vi "Receive Value Change Event.vi"(8 "error in (no error)":errorcluster, 10 "ValueChangeMsg":refnum<class "ValueChangeMsg.lvclass">, 11 "TwoButtonDialogBox in":refnum<class "TwoButtonDialogBox.lvclass">) -> (0 "error out":errorcluster, 3 "TwoButtonDialogBox out":refnum<class "TwoButtonDialogBox.lvclass">)   [LabVIEW 2017, in "TwoButtonDialogBox.lvlib" / "TwoButtonDialogBox.lvclass"]
doc: "<License>\nCopyright © 2017 Composed Systems, LLC | All rights reserved\nwww.composed.io\n\nAuthor: Ethan Stern <ethan.stern@composed.io>\n\nThis software is provided \"AS IS\" WITHOUT WARRANTIES, either express or implied, AND IS FOR EDUCATIONAL PURPOSES ONLY.\n</License>"
uses:
  TwoButtonDialogBox.lvclass
  C:/Program Files (x86)/National Instruments/LabVIEW 2017/vi.lib/ActorFramework/Actor/Actor.lvclass
  Framework/ActorEvents/IEventAggregator Messages/ValueChangeMsg/ValueChangeMsg.lvclass
  <vilib>/ActorFramework/Actor/Actor.lvclass/Actor.ctl
  <vilib>/ActorFramework/Message Enqueuer/Message Enqueuer.lvclass/Message Enqueuer.ctl
  Framework/ActorEvents/IEventAggregator Messages/ValueChangeMsg/ValueChangeMsg.lvclass/ValueChangeMsg.ctl
  TwoButtonDialogBox.lvclass/TwoButtonDialogBox.ctl
  <vilib>/ActorFramework/Message Enqueuer/Init from Existing Queue.vi
  <vilib>/ActorFramework/Message Enqueuer/Enqueue.vi
  <vilib>/ActorFramework/Stop Msg/Stop Msg.lvclass
  C:/Program Files (x86)/National Instruments/LabVIEW 2017/vi.lib/ActorFramework/Message/Message.lvclass
  <vilib>/ActorFramework/Message Priority Queue/Priority Enqueue.vi
  <vilib>/ActorFramework/Message Enqueuer/Message Enqueuer.lvclass
  Framework/IDialogBox/IDialogBox Messages/Dialog Return Msg/Dialog Return Msg.lvclass
  <vilib>/ActorFramework/Actor/Actor.lvclass
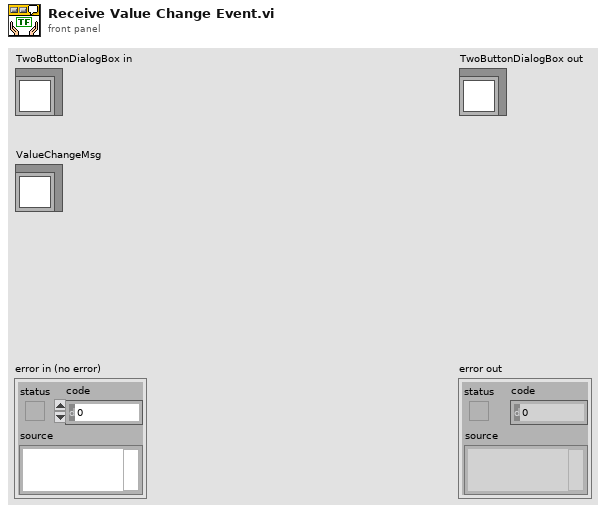
[diagram p1: front panel]
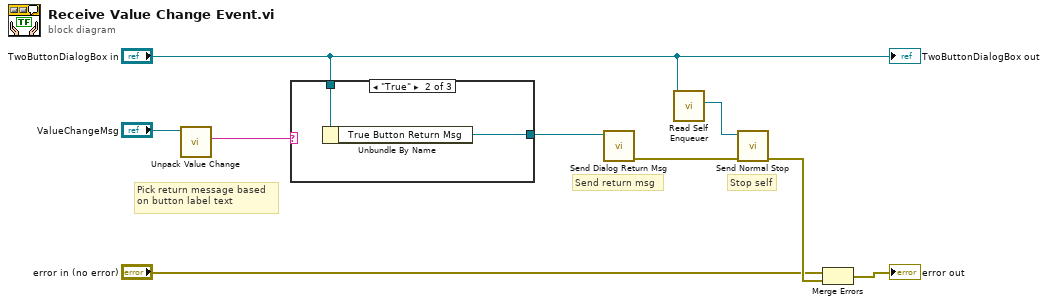
[diagram p0: block diagram]
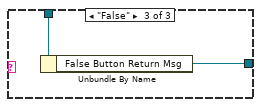
[diagram p3: hidden frame]
diagram:
  # "Pick return message based\non button label text"
  # "Stop self"
  # "Send return msg"
  n1 = call "Unpack Value Change.vi"("ValueChangeMsg"="ValueChangeMsg") -> ("Control Label"=w1:string)  [unwired: 6 in, 4 out]
  n2 = case shown="\"True\"" w1 {
    tunnel: [_ w11 w13] -> w2
    tunnel: "TwoButtonDialogBox in" -> [_ w10 w12]
    frame Default {
    }
    frame "True" {
      n3 = Unbundle By Name(w10) -> ("True Button Return Msg"=w11:refnum<class "Dialog Return Msg.lvclass">)
    }
    frame "False" {
      n4 = Unbundle By Name(w12) -> ("False Button Return Msg"=w13:refnum<class "Dialog Return Msg.lvclass">)
    }
  }
  n5 = call "Send Dialog Return Msg.vi"("Dialog Return Msg"=w2) -> ("error out"=w8:errorcluster)  [unwired: 10 in]
  n6 = call <vilib>:"Read Self Enqueuer.vi"("Actor"="TwoButtonDialogBox in") -> ("Self Enqueuer"=w9:refnum<class "Message Enqueuer.lvclass">)  [unwired: 10 in]
  n7 = call <vilib>:"Send Normal Stop.vi"("error in (no error)"=w8, "Message Enqueuer"=w9) -> ("error out"=w7:errorcluster)  [unwired: 9 in]
  n8 = Merge Errors("error in (no error)", w7) -> (→"error out":errorcluster)
  "TwoButtonDialogBox out" <- "TwoButtonDialogBox in"
